vi "Unloading.vi"(8 "error In":errorcluster) -> (0 "error out":errorcluster)   [LabVIEW 2017]
uses:
  <vilib>/Utility/error.llb/DialogType.ctl
  Controls/Unloading_Cyc_Data.ctl
  Controls/QUEUE_STATES.ctl
  Controls/Unload_St.ctl
  <vilib>/Utility/file.llb/Read Delimited Spreadsheet (string).vi
  Global/PLC_to_Auto.vi
  <vilib>/Instr/_visa.llb/VISA Configure Serial Port (Instr).vi
panel:
  out "qr scanned":bool=TRUE
  out "SELECTED Chld Part":T1
  out "Expected Code:":string
  out "DOOR NO.":string
  out "output cluster":cluster{"Feeder Door Open":bool, "Address":u16}
  out "raw scan code":string
  in  "Boolean":bool
  in  "String":string
  out "Bins/Box":i32
  out "Scanner Comm":bool
  out "Stop scanner":bool
  out "CYCLE STATUS":string
  out "CURRENT PLAN":T2
  out "SCAN CODE:":string
  out "Selected Plan structure":string[][](table)
  out "Plan Selected:":string
  out "USER:-":string
  in  "Stop":bool
  out "DATE/TIME":string
  out "Screen Name":string
  # "DOOR NUMBER"
  # "BIN STATUS"
  # "DOOR NUMBER"
  # "BIN STATUS"
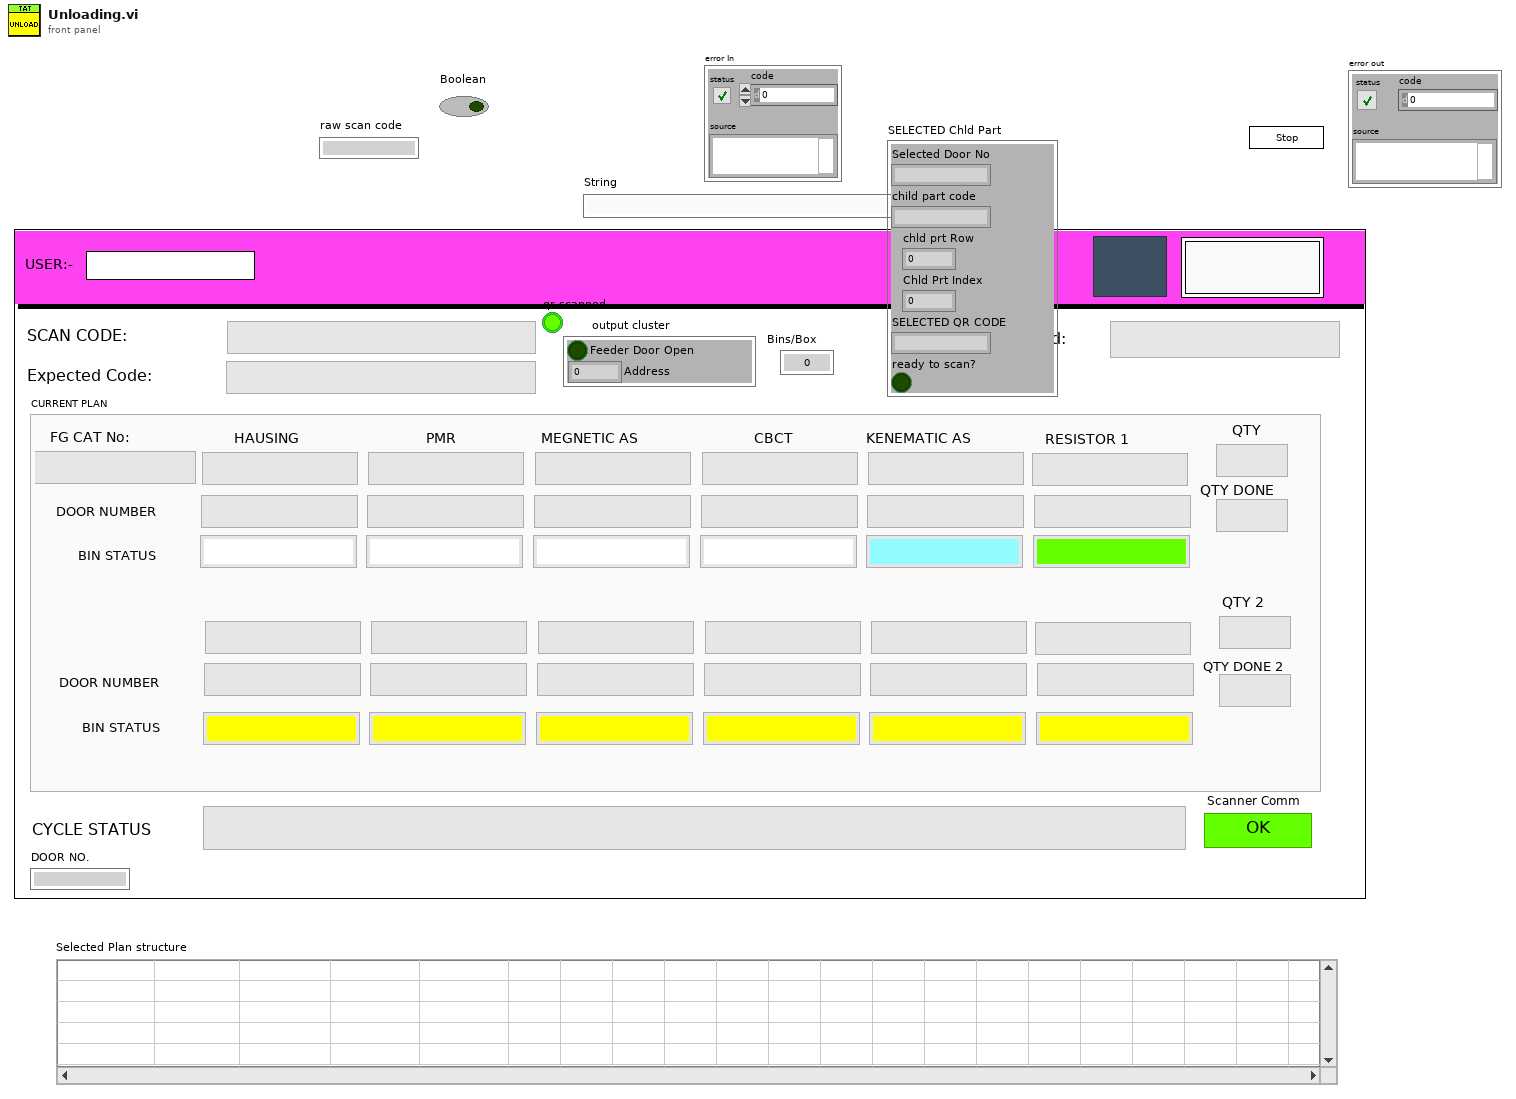
[diagram p1: front panel]
types:
  T1 = cluster{"Selected Door No":string, "child part code":string, "chld prt Row":i32, "Chld Prt Index":i32, "SELECTED QR CODE":string, "ready to scan?":bool}
  T2 = cluster{"FG CAT No:":string, "HAUSING":string, "PMR":string, "MEGNETIC AS":string, "CBCT":string, "KENEMATIC AS":string, "RESISTOR 1":string, "HAUSING DOOR":string, "PMR DOOR":string, "MAGNETIC AS DOOR":string, "CBCT DOOR":string, "KINEMATIC AS DOOR":string, "RESISTOR 1 DOOR":string, "HAUSING FEED STATUS":string, "PMR FEED STATUS":string, "MAGNETIC AS FEEED STATUS":string, "CBCT FEED STATUS":string, "KINEMATIC AS FEED STATUS":string, "RESISTOR 1 FEED STATUS":string, "QTY":string, "QTY DONE":string, "HAUSING 2":string, "PMR 2":string, "MEGNETIC AS 2":string, "CBCT 2":string, "KENEMATIC AS 2":string, "RESISTOR 2":string, "HAUSING DOOR 2":string, "PMR DOOR 2":string, "MAGNETIC AS DOOR 2":string, "CBCT DOOR 2":string, "KINEMATIC AS DOOR 2":string, "RESISTOR 1 DOOR 2":string, "HAUSING FEED STATUS 2":string, "PMR FEED STATUS 2":string, "MAGNETIC AS FEEED STATUS 2":string, "CBCT FEED STATUS 2":string, "KINEMATIC AS FEED STATUS 2":string, "RESISTOR 1 FEED STATUS 2":string, "QTY 2":string, "QTY DONE 2":string}
  T3 = typedef "Unloading_Cyc_Data.ctl" = cluster{"Cycle_Plan":path, "Plan_Data":string[][], "Scanned_Data":string[], "SELECTED Chld Part":cluster{"Selected Door No":string, "child part code":string, "chld prt Row":i32, "Chld Prt Index":i32, "EXPECTED QR CODE":string, "ready to scan?":bool}, "feed Status Indi":refnum<vi>[], "Recipe Selected":cluster{"Bin/Box Mode":i32, "Selected Section":i32}, "ALL CSV DATA":string[][]}
  T4 = typedef "DialogType.ctl" = u16
  T5 = enum32{"invalid app kind", "Development System", "Run Time System", "Student Edition", "Embedded LabVIEW", "Evaluation", "Custom"}
  T6 = typedef "QUEUE_STATES.ctl" = enum16{"CREATE Q", "EN Q", "DE Q", "CLOSE Q"}
  T7 = cluster{"Printer IP":string, "PLC IP Address":string, "Scanner Com":refnum<visa-resource-name>}
  T8 = typedef "Unload_St.ctl" = enum16{"Package_Qty_Count", "GENERATE_QR_PRNT", "Cluster_update", "Read_Plan", "QR_Scanned", "Int", "Chk_Previous_State", "Chk_Loaded_and_Open_Door", "Update_Plan_Cluster", "Error_Handler", "Wait", "Close_Door", "Stop"}
  T9 = cluster{"Selected Door No":string, "child part code":string, "chld prt Row":i32, "Chld Prt Index":i32, "EXPECTED QR CODE":string, "ready to scan?":bool}
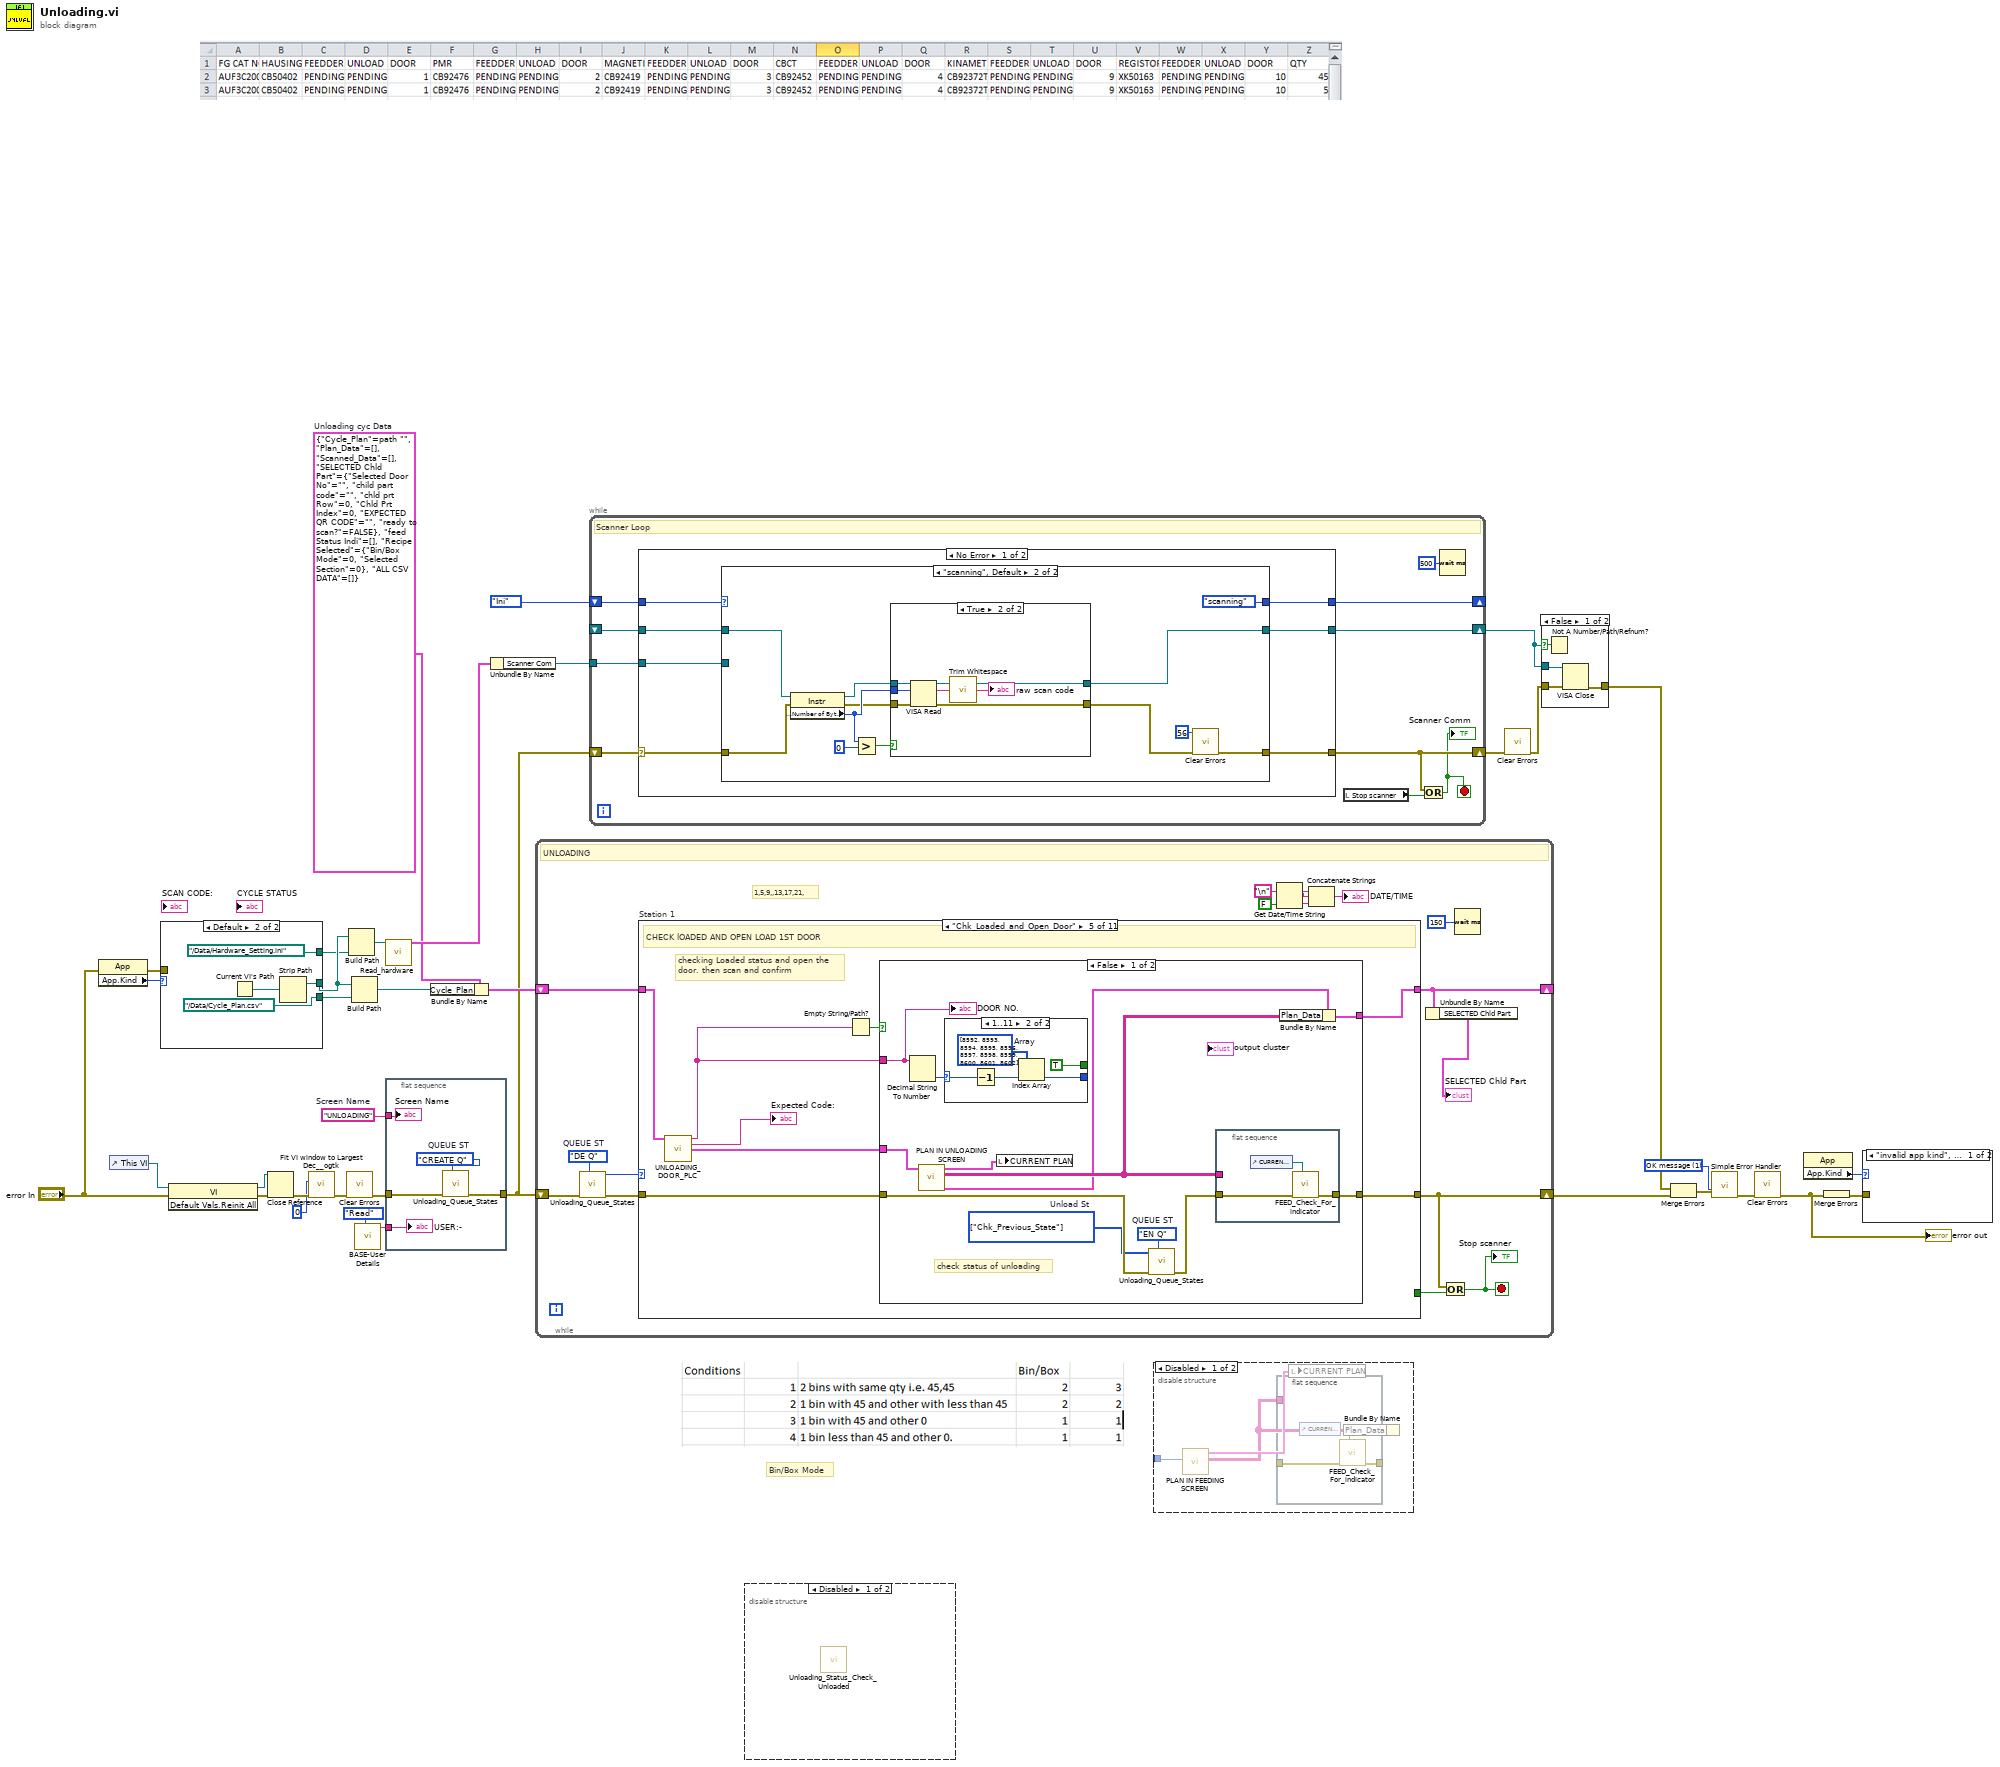
[diagram p0: block diagram]
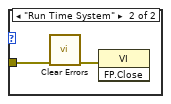
[diagram p3: hidden frame]
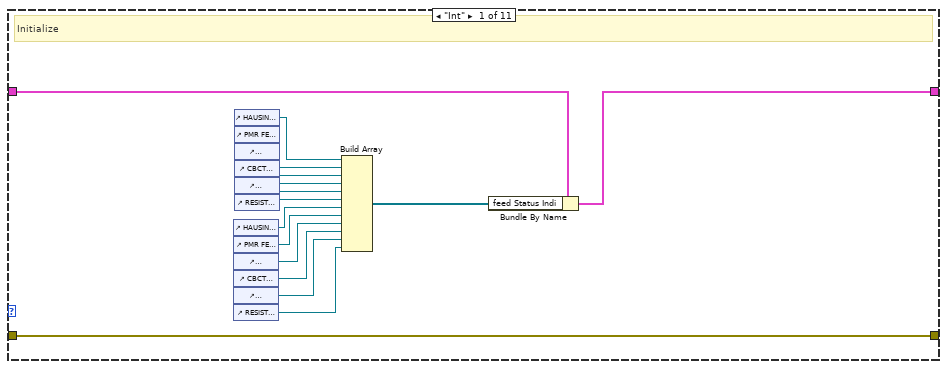
[diagram p4: hidden frame]
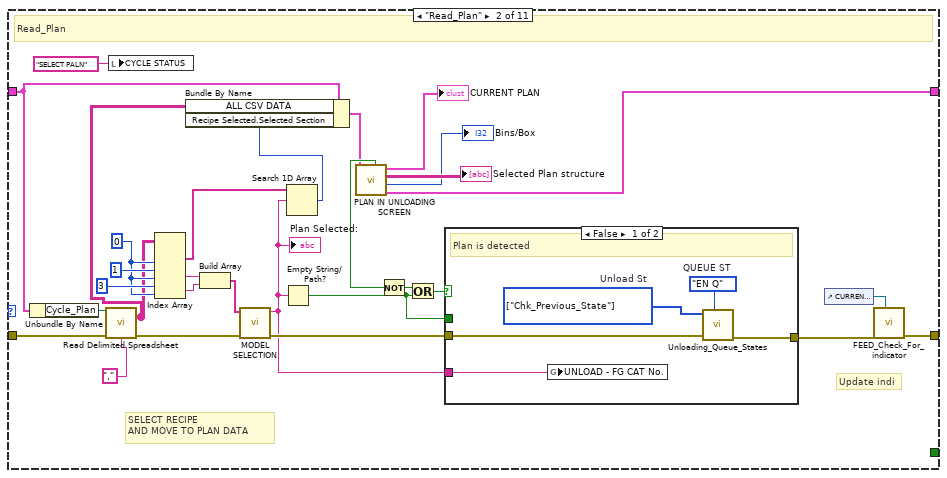
[diagram p5: hidden frame]
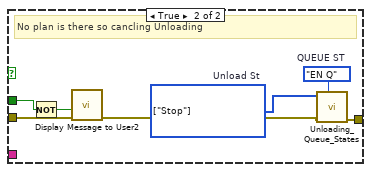
[diagram p6: hidden frame]
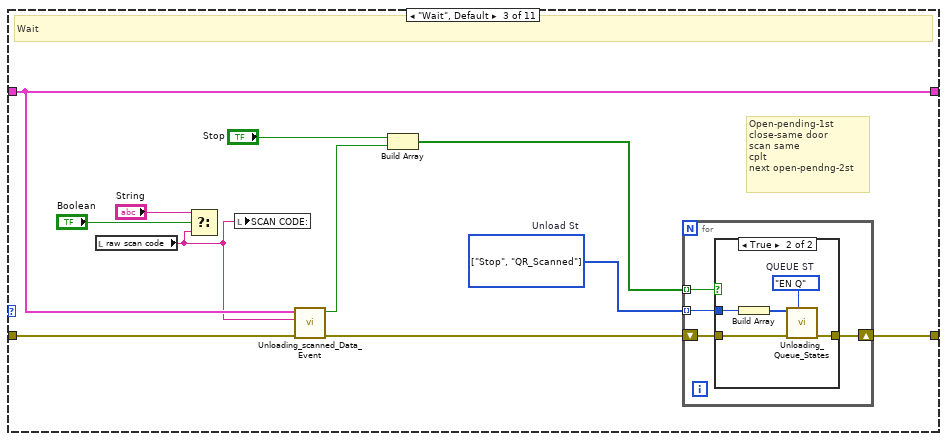
[diagram p7: hidden frame]
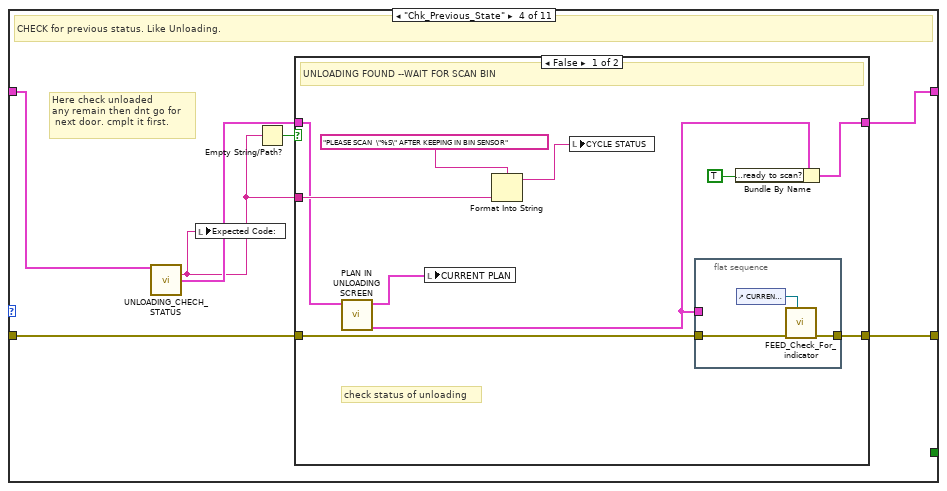
[diagram p9: hidden frame]
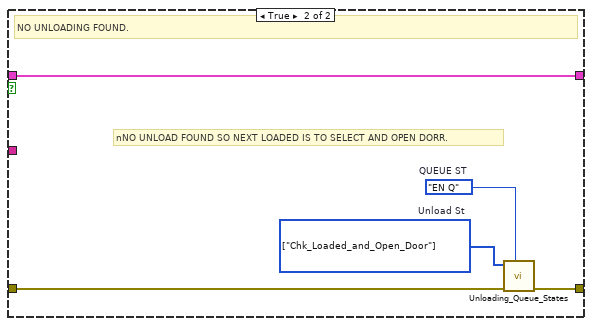
[diagram p10: hidden frame]
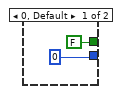
[diagram p11: hidden frame]
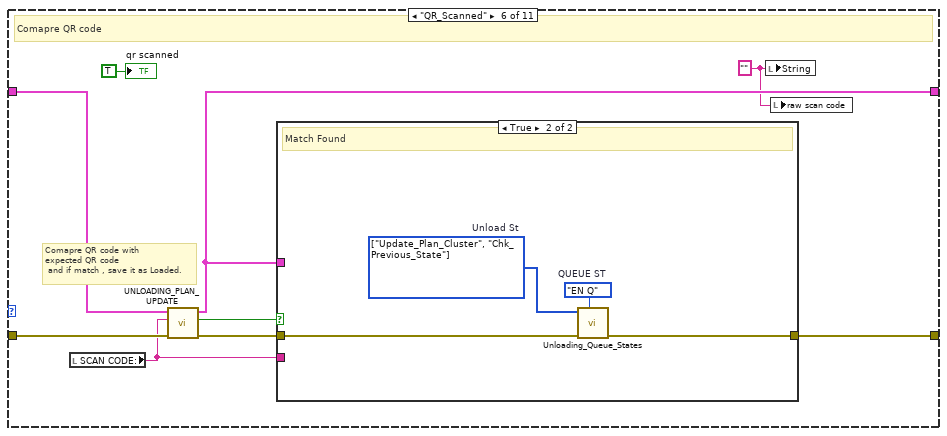
[diagram p13: hidden frame]
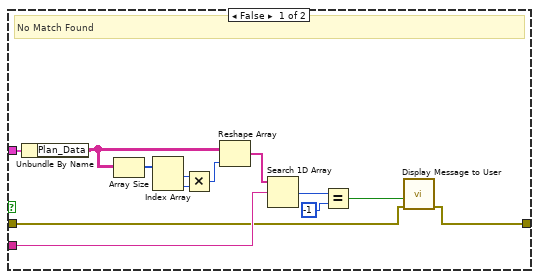
[diagram p14: hidden frame]
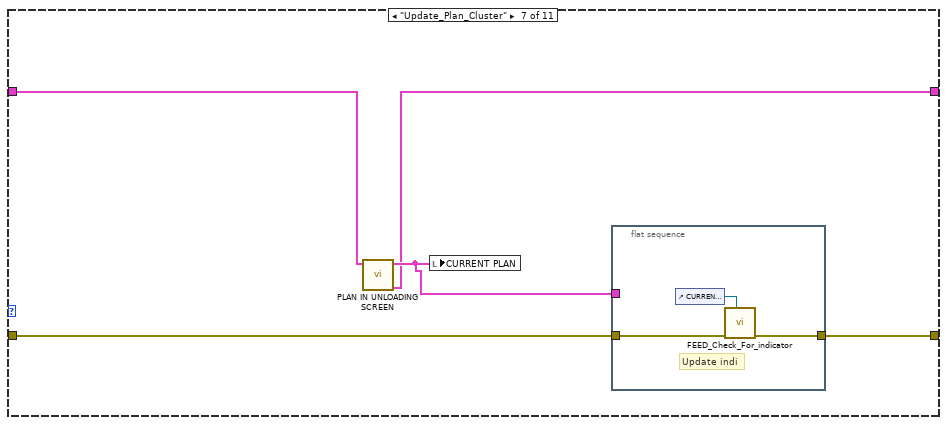
[diagram p15: hidden frame]
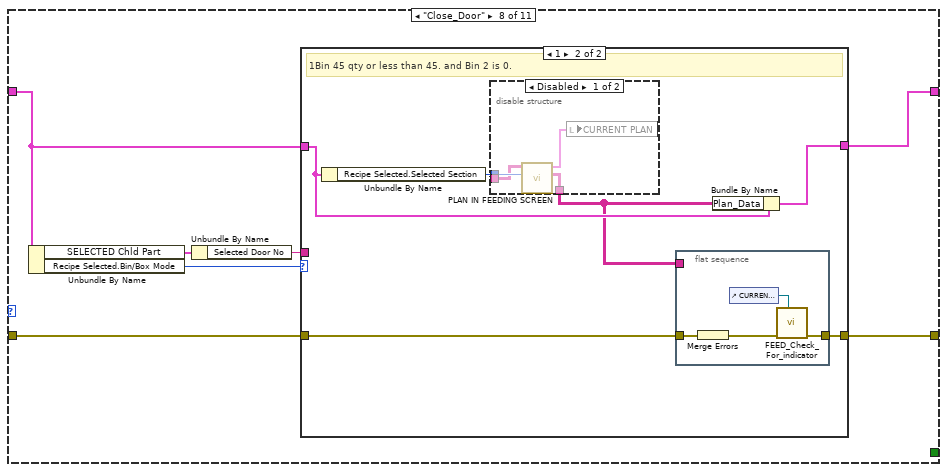
[diagram p16: hidden frame]
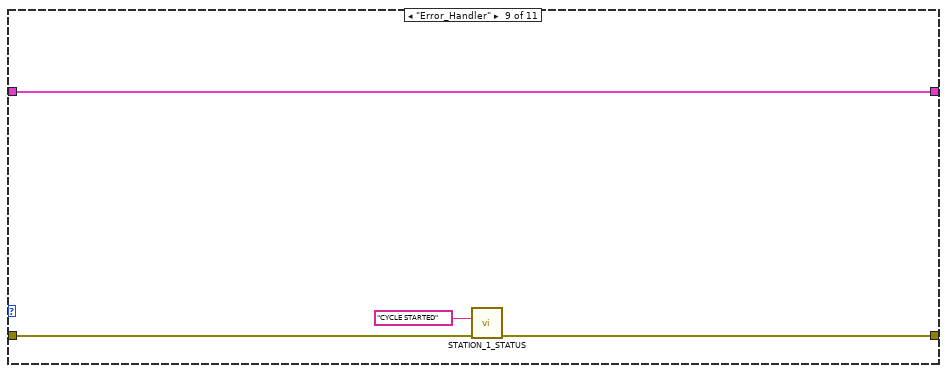
[diagram p19: hidden frame]
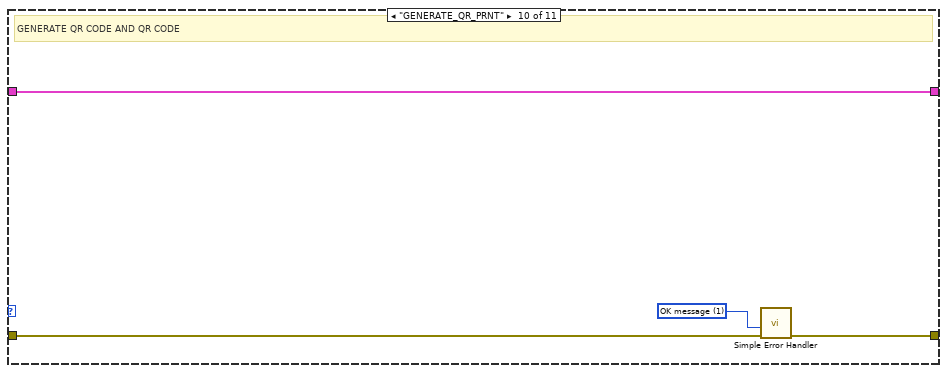
[diagram p20: hidden frame]
diagram:
  w1 = T3 {"Cycle_Plan"=path "", "Plan_Data"=[], "Scanned_Data"=[], "SELECTED Chld Part"={"Selected Door No"="", "child part code"="", "chld prt Row"=0, "Chld Prt Index"=0, "EXPECTED QR CODE"="", "ready to scan?"=FALSE}, "feed Status Indi"=[], "Recipe Selected"={"Bin/Box Mode"=0, "Selected Section"=0}, "ALL CSV DATA"=[]}  # Unloading cyc Data
  w18 = "UNLOADING"  # Screen Name
  w29 = T4 1 items=["no dialog", "OK message", "continue or stop message", "OK message + warnings", "continue/stop + warnings"] ("type of dialog (OK msg:1)")
  # "Bin/Box Mode"
  n1 = property class="App"(error in="error In") -> (error out=w25:errorcluster, "App.Kind"=w27:T5)  [unwired: 1 in, 1 out]
  n2 = control-ref of="This VI"() -> (w36:refnum<vi>)
  n3 = case shown="Default" w27 {
    tunnel: [path "Data/Cycle_Plan.csv" ("path") path "../Data/Cycle_Plan.csv" ("path")] -> w26
    tunnel: [w37 w41] -> w7
    tunnel: w25 -> [_ _]
    tunnel: [path "Data/Hardware_Setting.ini" ("path") path "../Data/Hardware_Setting.ini" ("path")] -> w6
    frame "Run Time System" {
      n4 = call <vilib>:"Application Directory.vi"() -> ("Application Directory"=w37:path)
    }
    frame Default {
      n5 = Current VI's Path() -> (path=w42:path)
      n6 = Strip Path(path=w42) -> (stripped path=w41:path)  [unwired: 1 out]
    }
  }
  n7 = invoke class="VI" method="Default Vals.Reinit All"(reference=w36, error in="error In") -> (reference out=w34:refnum<vi>, error out=w35:errorcluster)  [unwired: 1 in, 1 out]
  n8 = Close Reference(reference=w34, error in (no error)=w35) -> (error out=w33:errorcluster)
  n9 = call <userlib>:"Fit VI window to Largest Dec__ogtk.vi"("error in (no error)"=w33, "border spacing (2 px)"=0) -> ("error out"=w23:errorcluster)  [unwired: 4 in, 1 out]
  n10 = call <vilib>:"Clear Errors.vi"("error in (no error)"=w23) -> ("error out"=w11:errorcluster)  [unwired: 5 in, 1 out]
  n11 = Build Path(base path=w7, name or relative path=w6) -> (appended path=w5:path)
  n12 = Build Path(base path=w7, name or relative path=w26) -> (appended path=w20:path)
  n13 = call "BASE-User Details.vi"("Enum"=enum16{"Read", "Write"}."Read") -> ("User Name Out"=w30:string)  [unwired: 9 in, 1 out]
  n14 = flat-sequence {
    tunnel: [w45] -> w12
    tunnel: w11 -> [w46]
    tunnel: w30 -> [w48]
    tunnel: w18 -> [w47]
    frame #0 {
      w44 = QUEUE_STATES."CREATE Q"  # QUEUE ST
      n15 = call "Unloading_Queue_States.vi"("QUEUE ST"=w44, "error in"=w46) -> ("error OUT"=w45:errorcluster)  [unwired: 8 in, 1 out]
      "USER:-" <- w48
      "Screen Name" <- w47
    }
  }
  n16 = call "Read_hardware.vi"("configuration file path"=w5) -> ("data"=w9:T7)  [unwired: 10 in]
  n17 = Bundle By Name(cluster=w1, "Cycle_Plan"=w20) -> (w19:T3)
  n18 = Unbundle By Name(w9) -> ("Scanner Com"=w8:refnum<visa-resource-name>)
  n19 = while {
    shift-right: [w50] -> _
    shift-left: w19 -> [w57]
    shift-right: [w55] -> w10
    shift-left: w12 -> [w54]
    stop <- w56 stop-if-true
    w52 = QUEUE_STATES."DE Q"  # QUEUE ST
    # "1,5,9,,13,17,21,"
    # "UNLOADING"
    n20 = call "Unloading_Queue_States.vi"("QUEUE ST"=w52, "error in"=w54) -> ("error OUT"=w53:errorcluster, "Unload ST"=w51:T8)  [unwired: 8 in]
    n21 = case "Station 1" shown="\"Chk_Loaded_and_Open_Door\"" w51 {
      tunnel: [_ _ _ _ _ _ _ _ _ _ TRUE] -> w58
      tunnel: [w80 w97 w130 w148 w173 w205 w229 w239 w258 w263 w265] -> w55
      tunnel: w53 -> [w80 w108 w124 w147 w172 w208 w230 w240 w259 w262 w269]
      tunnel: w57 -> [w67 w82 w126 w143 w169 w207 w227 w236 w257 w261 w268]
      tunnel: [w66 w81 w126 w146 w170 w203 w226 w235 w257 w261 w268] -> w50
      frame "Int" {
        # "Initialize"
        n22 = control-ref of="HAUSING FEED STATUS 2"() -> (w74:refnum<vi>)
        n23 = control-ref of="PMR FEED STATUS 2"() -> (w75:refnum<vi>)
        n24 = control-ref of="MAGNETIC AS FEEED STATUS 2"() -> (w76:refnum<vi>)
        n25 = control-ref of="CBCT FEED STATUS 2"() -> (w77:refnum<vi>)
        n26 = control-ref of="KINEMATIC AS FEED STATUS 2"() -> (w78:refnum<vi>)
        n27 = control-ref of="RESISTOR 1 FEED STATUS 2"() -> (w79:refnum<vi>)
        n28 = control-ref of="HAUSING FEED STATUS"() -> (w68:refnum<vi>)
        n29 = control-ref of="PMR FEED STATUS"() -> (w69:refnum<vi>)
        n30 = control-ref of="MAGNETIC AS FEEED STATUS"() -> (w70:refnum<vi>)
        n31 = control-ref of="CBCT FEED STATUS"() -> (w71:refnum<vi>)
        n32 = control-ref of="KINEMATIC AS FEED STATUS"() -> (w72:refnum<vi>)
        n33 = control-ref of="RESISTOR 1 FEED STATUS"() -> (w73:refnum<vi>)
        n34 = Build Array(w68, w69, w70, w71, w72, w73, w74, w75, w76, w77, w78, w79) -> (w65:refnum<vi>[])
        n35 = Bundle By Name(cluster=w67, "feed Status Indi"=w65) -> (w66:T3)
      }
      frame "Read_Plan" {
        w100 = 0
        # "SELECT RECIPE\nAND MOVE TO PLAN DATA"
        # "Update indi"
        # "Read_Plan"
        n36 = Unbundle By Name(w82) -> ("Cycle_Plan"=w107:path)
        n37 = call-poly <vilib>:"Read Delimited Spreadsheet.vi"("file path (dialog if empty)"=w107, "error in (no error)"=w108, "delimiter (\\t)"=",") -> ("all rows"=w83:string[][], "error out"=w101:errorcluster)  [unwired: 7 in, 4 out]
        n38 = local write "CYCLE STATUS"("SELECT PALN") -> ()
        n39 = Index Array(array=w83, index (col) #1=w100, index (row) #2=1, index (col) #2=w100, index (row) #3=3, index (col) #3=w100) -> (element #1=w99:string[], element #2=w104:string, element #3=w103:string)  [unwired: 1 in]
        n40 = Build Array(w104, w103) -> (w102:string[])
        n41 = call "MODEL SELECTION.vi"("error in (no error)"=w101, "Plan List"=w102) -> ("error out 2"=w95:errorcluster, "Plan Selected"=w87:string)  [unwired: 7 in, 1 out]
        "Plan Selected:" <- w87
        n42 = Empty String/Path?(string/path=w87) -> (empty?=w91:bool)
        n43 = Search 1D Array(1D array=w99, element=w87) -> (index of element=w85:i32)  [unwired: 1 in]
        n44 = Bundle By Name(cluster=w82, "ALL CSV DATA"=w83, "Recipe Selected.Selected Section"=w85) -> (w84:T3)
        n45 = call "PLAN IN UNLOADING SCREEN.vi"("Unloading cyc Data"=w84) -> ("Unloading cyc Data 2"=w81:T3, "Bin/Box"=→"Bins/Box":i32, "PLAN DATA Out"=→"Selected Plan structure":string[][], "CURRENT PLAN"=→"CURRENT PLAN":T2, "FEED CMPLT?"=w93:bool)  [unwired: 6 in]
        n46 = Not(x=w93) -> (.not. x?=w92:bool)
        n47 = Or(x=w92, y=w91) -> (x .or. y?=w94:bool)
        n48 = case shown="False" w94 {
          tunnel: w95 -> [w114 w119]
          tunnel: [w113 w120] -> w98
          tunnel: w91 -> [_ w117]
          tunnel: w87 -> [w110 _]
          frame False {
            w111 = T8[] [enum."Chk_Previous_State"] items=["Package_Qty_Count", "GENERATE_QR_PRNT", "Cluster_update", "Read_Plan", "QR_Scanned", "Int", "Chk_Previous_State", "Chk_Loaded_and_Open_Door", "Update_Plan_Cluster", "Error_Handler", "Wait", "Close_Door", "Stop"]  # Unload St
            w112 = QUEUE_STATES."EN Q"  # QUEUE ST
            # "Plan is detected"
            n49 = global write "PLC_to_Auto.vi" "UNLOAD - FG CAT No."(w110) -> ()
            n50 = call "Unloading_Queue_States.vi"("QUEUE ST"=w112, "error in"=w114, "Unload St"=w111) -> ("error OUT"=w113:errorcluster)  [unwired: 7 in, 1 out]
          }
          frame True {
            w115 = T8[] [enum."Stop"] items=["Package_Qty_Count", "GENERATE_QR_PRNT", "Cluster_update", "Read_Plan", "QR_Scanned", "Int", "Chk_Previous_State", "Chk_Loaded_and_Open_Door", "Update_Plan_Cluster", "Error_Handler", "Wait", "Close_Door", "Stop"]  # Unload St
            w121 = QUEUE_STATES."EN Q"  # QUEUE ST
            # "No plan is there so cancling Unloading"
            n51 = Not(x=w117) -> (.not. x?=w116:bool)
            n52 = call "Display Message to User2"("error in (no error)"=w119, "Enable"=w116) -> ("error out"=w118:errorcluster)  [unwired: 8 in, 1 out]
            n53 = call "Unloading_Queue_States.vi"("QUEUE ST"=w121, "error in"=w118, "Unload St"=w115) -> ("error OUT"=w120:errorcluster)  [unwired: 7 in, 1 out]
          }
        }
        n54 = control-ref of="CURRENT PLAN"() -> (w96:refnum<vi>)
        n55 = call "FEED_Check_For_indicator.vi"("CURRENT PLAN"=w96, "error in (no error)"=w98) -> ("error out"=w97:errorcluster)  [unwired: 9 in]
      }
      frame "Wait", Default {
        w127 = T8[] [enum."Stop", enum."QR_Scanned"] items=["Package_Qty_Count", "GENERATE_QR_PRNT", "Cluster_update", "Read_Plan", "QR_Scanned", "Int", "Chk_Previous_State", "Chk_Loaded_and_Open_Door", "Update_Plan_Cluster", "Error_Handler", "Wait", "Close_Door", "Stop"]  # Unload St
        # "Open-pending-1st\nclose-same door\nscan same\ncplt\nnext open-pendng-2st"
        # "Wait"
        n56 = local read "raw scan code"() -> (w122:string)
        n57 = Select(t="String", s="Boolean", f=w122) -> ()  [unwired: 1 out]
        n58 = local write "SCAN CODE:"(w122) -> ()
        n59 = call "Unloading_scanned_Data_Event.vi"("Unloading cyc Data"=w126, "Scanned  Data"=w122, "error in"=w124) -> ("Scanned ?"=w125:bool, "error out"=w123:errorcluster)  [unwired: 6 in]
        n60 = Build Array("Stop", w125) -> (w128:bool[])
        n61 = for {
          shift-right: [w135] -> w130
          shift-left: w123 -> [w136]
          tunnel: w128 -> [w134] mode=indexing
          tunnel: w127 -> [w133] mode=indexing
          n62 = case shown="True" w134 {
            tunnel: w136 -> [w137 w141]
            tunnel: [w137 w140] -> w135
            tunnel: w133 -> [_ w139]
            frame False {
            }
            frame True {
              w142 = QUEUE_STATES."EN Q"  # QUEUE ST
              n63 = Build Array(w139) -> (w138:T8[])
              n64 = call "Unloading_Queue_States.vi"("QUEUE ST"=w142, "error in"=w141, "Unload St"=w138) -> ("error OUT"=w140:errorcluster)  [unwired: 7 in, 1 out]
            }
          }
        }
      }
      frame "Chk_Previous_State" {
        # "Here check unloaded\nany remain then dnt go for\n next door. cmplt it first."
        # "CHECK for previous status. Like Unloading."
        n65 = call "UNLOADING_CHECH_STATUS.vi"("Unloading cyc Data"=w143) -> ("QR Code"=w144:string, "Unloading cyc Data OUT"=w145:T3)  [unwired: 12 in, 1 out]
        n66 = local write "Expected Code:"(w144) -> ()
        n67 = Empty String/Path?(string/path=w144) -> (empty?=w149:bool)
        n68 = case shown="False" w149 {
          tunnel: [w158 w165] -> w148
          tunnel: w147 -> [w159 w166]
          tunnel: w145 -> [w150 w167]
          tunnel: [w156 w167] -> w146
          tunnel: w144 -> [w154 _]
          frame False {
            # "check status of unloading"
            # "UNLOADING FOUND --WAIT FOR SCAN BIN"
            n69 = call "PLAN IN UNLOADING SCREEN.vi"("Unloading cyc Data"=w150) -> ("Unloading cyc Data 2"=w151:T3, "CURRENT PLAN"=w157:T2)  [unwired: 6 in, 3 out]
            n70 = local write "CURRENT PLAN"(w157) -> ()
            n71 = Format Into String(format string="PLEASE SCAN  \"%S\" AFTER KEEPING IN BIN SENSOR", w154) -> (resulting string=w153:string)  [unwired: 2 in, 1 out]
            n72 = local write "CYCLE STATUS"(w153) -> ()
            n73 = flat-sequence {
              tunnel: w159 -> [w161]
              tunnel: [w160] -> w158
              tunnel: w151 -> [_]
              frame #0 {
                n74 = control-ref of="CURRENT PLAN"() -> (w162:refnum<vi>)
                n75 = call "FEED_Check_For_indicator.vi"("CURRENT PLAN"=w162, "error in (no error)"=w161) -> ("error out"=w160:errorcluster)  [unwired: 9 in]
              }
            }
            n76 = Bundle By Name(cluster=w151, "SELECTED Chld Part.ready to scan?"=TRUE) -> (w156:T3)
          }
          frame True {
            w163 = T8[] [enum."Chk_Loaded_and_Open_Door"] items=["Package_Qty_Count", "GENERATE_QR_PRNT", "Cluster_update", "Read_Plan", "QR_Scanned", "Int", "Chk_Previous_State", "Chk_Loaded_and_Open_Door", "Update_Plan_Cluster", "Error_Handler", "Wait", "Close_Door", "Stop"]  # Unload St
            w164 = QUEUE_STATES."EN Q"  # QUEUE ST
            # "nNO UNLOAD FOUND SO NEXT LOADED IS TO SELECT AND OPEN DORR."
            # "NO UNLOADING FOUND."
            n77 = call "Unloading_Queue_States.vi"("QUEUE ST"=w164, "error in"=w166, "Unload St"=w163) -> ("error OUT"=w165:errorcluster)  [unwired: 7 in, 1 out]
          }
        }
      }
      frame "Chk_Loaded_and_Open_Door" {
        # "checking Loaded status and open the\ndoor. then scan and confirm"
        # "CHECK lOADED AND OPEN LOAD 1ST DOOR"
        n78 = call "UNLOADING_DOOR_PLC.vi"("Unloading cyc Data"=w169) -> ("DOOR NO."=w175:string, "QR Code"=→"Expected Code:":string, "Unloading cyc Data 2"=w168:T3)  [unwired: 11 in, 1 out]
        n79 = Empty String/Path?(string/path=w175) -> (empty?=w174:bool)
        n80 = case shown="False" w174 {
          tunnel: w175 -> [w186 _]
          tunnel: [w185 w199] -> w173
          tunnel: w172 -> [w179 w199]
          tunnel: [w182 w198] -> w170
          tunnel: w168 -> [w181 w198]
          frame False {
            w177 = T8[] [enum."Chk_Previous_State"] items=["Package_Qty_Count", "GENERATE_QR_PRNT", "Cluster_update", "Read_Plan", "QR_Scanned", "Int", "Chk_Previous_State", "Chk_Loaded_and_Open_Door", "Update_Plan_Cluster", "Error_Handler", "Wait", "Close_Door", "Stop"]  # Unload St
            w180 = QUEUE_STATES."EN Q"  # QUEUE ST
            # "check status of unloading"
            n81 = Decimal String To Number(string=w186) -> (number=w187:i32)  [unwired: 2 in, 1 out]
            n82 = call "PLAN IN UNLOADING SCREEN.vi"("Unloading cyc Data"=w181) -> ("Unloading cyc Data 2"=w176:T3, "PLAN DATA Out"=w183:string[][], "CURRENT PLAN"=w184:T2)  [unwired: 6 in, 2 out]
            n83 = case shown="1..11" w187 {
              selector: w187 -> [_ w197]
              tunnel: [u16 0 w196] -> _
              tunnel: [FALSE TRUE] -> _
              frame 0, Default {
              }
              frame 1..11 {
                w194 = i32[] [8592, 8593, 8594, 8595, 8596, 8597, 8598, 8599, 8600, 8601, 8602]  # Array
                n84 = Decrement(x=w197) -> (x-1=w193:i32)
                n85 = Index Array(array=w194, index=w193) -> (element=w196:i32)
              }
            }
            n86 = local write "CURRENT PLAN"(w184) -> ()
            n87 = call "Unloading_Queue_States.vi"("QUEUE ST"=w180, "error in"=w179, "Unload St"=w177) -> ("error OUT"=w178:errorcluster)  [unwired: 7 in, 1 out]
            n88 = flat-sequence {
              tunnel: w178 -> [w189]
              tunnel: [w188] -> w185
              tunnel: w183 -> [_]
              frame #0 {
                n89 = control-ref of="CURRENT PLAN"() -> (w190:refnum<vi>)
                n90 = call "FEED_Check_For_indicator.vi"("CURRENT PLAN"=w190, "error in (no error)"=w189) -> ("error out"=w188:errorcluster)  [unwired: 9 in]
              }
            }
            n91 = Bundle By Name(cluster=w176, "Plan_Data"=w183) -> (w182:T3)
            "DOOR NO." <- w186
          }
          frame True {
          }
        }
      }
      frame "QR_Scanned" {
        w200 = ""
        # "Comapre QR code with \nexpected QR code\n and if match , save it as Loaded."
        # "Comapre QR code"
        n92 = local read "SCAN CODE:"() -> (w202:string)
        n93 = call "UNLOADING_PLAN_UPDATE.vi"("error in (no error)"=w208, "SCAN CODE:"=w202, "Unloading cyc Data in"=w207) -> ("error out"=w206:errorcluster, "QR Match ?"=w204:bool, "Unloading cyc Data out"=w203:T3)  [unwired: 6 in]
        n94 = case shown="True" w204 {
          tunnel: w206 -> [w210 w224]
          tunnel: [w209 w223] -> w205
          tunnel: w203 -> [w221 _]
          tunnel: w202 -> [w214 _]
          frame False {
            # "No Match Found"
            n95 = Unbundle By Name(w221) -> ("Plan_Data"=w216:string[][])
            n96 = Array Size(array=w216) -> (size(s)=w220:i32[])
            n97 = Index Array(array=w220) -> (element #1=w218:i32, element #2=w219:i32)  [unwired: 2 in]
            n98 = Multiply(x=w218, y=w219) -> (x*y=w217:i32)
            n99 = Reshape Array(w216, w217) -> (w215:string[])
            n100 = Search 1D Array(1D array=w215, element=w214) -> (index of element=w213:i32)  [unwired: 1 in]
            n101 = Equal?(x=w213, y=-1) -> (x = y?=w211:bool)
            n102 = call "Display Message to User"("error in (no error)"=w210, "Enable"=w211) -> ("error out"=w209:errorcluster)  [unwired: 8 in, 1 out]
          }
          frame True {
            w222 = T8[] [enum."Update_Plan_Cluster", enum."Chk_Previous_State"] items=["Package_Qty_Count", "GENERATE_QR_PRNT", "Cluster_update", "Read_Plan", "QR_Scanned", "Int", "Chk_Previous_State", "Chk_Loaded_and_Open_Door", "Update_Plan_Cluster", "Error_Handler", "Wait", "Close_Door", "Stop"]  # Unload St
            w225 = QUEUE_STATES."EN Q"  # QUEUE ST
            # "Match Found"
            n103 = call "Unloading_Queue_States.vi"("QUEUE ST"=w225, "error in"=w224, "Unload St"=w222) -> ("error OUT"=w223:errorcluster)  [unwired: 7 in, 1 out]
          }
        }
        n104 = local write "String"(w200) -> ()
        n105 = local write "raw scan code"(w200) -> ()
        "qr scanned" <- TRUE
      }
      frame "Update_Plan_Cluster" {
        n106 = call "PLAN IN UNLOADING SCREEN.vi"("Unloading cyc Data"=w227) -> ("Unloading cyc Data 2"=w226:T3, "CURRENT PLAN"=w228:T2)  [unwired: 6 in, 3 out]
        n107 = local write "CURRENT PLAN"(w228) -> ()
        n108 = flat-sequence {
          tunnel: w230 -> [w232]
          tunnel: [w231] -> w229
          tunnel: w228 -> [_]
          frame #0 {
            # "Update indi"
            n109 = control-ref of="CURRENT PLAN"() -> (w233:refnum<vi>)
            n110 = call "FEED_Check_For_indicator.vi"("CURRENT PLAN"=w233, "error in (no error)"=w232) -> ("error out"=w231:errorcluster)  [unwired: 9 in]
          }
        }
      }
      frame "Close_Door" {
        n111 = Unbundle By Name(w236) -> ("SELECTED Chld Part"=w237:T9, "Recipe Selected.Bin/Box Mode"=w234:i32)
        n112 = Unbundle By Name(w237) -> ("Selected Door No"=w238:string)
        n113 = case shown="1" w234 {
          tunnel: w240 -> [w241 w248]
          tunnel: [w241 w245] -> w239
          tunnel: w238 -> [_ _]
          tunnel: w236 -> [w242 w246]
          tunnel: [w242 w243] -> w235
          frame 0, Default {
          }
          frame 1 {
            # "1Bin 45 qty or less than 45. and Bin 2 is 0."
            n114 = Unbundle By Name(w246) -> ("Recipe Selected.Selected Section"=w247:i32)
            n115 = disable-structure shown="Disabled" {
              disable-tunnel: w247 -> [w252 _]
              disable-tunnel: _ -> [w250 _]
              disable-tunnel: [w249 _] -> w244
              frame Disabled {
                n116 = call "PLAN IN FEEDING SCREEN.vi"("Section selected"=w252, "PLAN In"=w250) -> ("PLAN Out"=w249:string[][], "CURRENT PLAN"=w251:T2)  [unwired: 6 in, 2 out]
                n117 = local write "CURRENT PLAN"(w251) -> ()
              }
              frame Enabled {
              }
            }
            n118 = flat-sequence {
              tunnel: w248 -> [w256]
              tunnel: [w253] -> w245
              tunnel: w244 -> [_]
              frame #0 {
                n119 = Merge Errors(w256) -> (w254:errorcluster)
                n120 = control-ref of="CURRENT PLAN"() -> (w255:refnum<vi>)
                n121 = call "FEED_Check_For_indicator.vi"("CURRENT PLAN"=w255, "error in (no error)"=w254) -> ("error out"=w253:errorcluster)  [unwired: 9 in]
              }
            }
            n122 = Bundle By Name(cluster=w246, "Plan_Data"=w244) -> (w243:T3)
          }
        }
      }
      frame "Error_Handler" {
        n123 = call "STATION_1_STATUS.vi"("error in (no error)"=w259, "STATUS"="CYCLE STARTED" ("Cycle Status")) -> ("error out"=w258:errorcluster)  [unwired: 9 in]
      }
      frame "GENERATE_QR_PRNT" {
        w264 = T4 1 items=["no dialog", "OK message", "continue or stop message", "OK message + warnings", "continue/stop + warnings"] ("type of dialog (OK msg:1)")
        # "GENERATE QR CODE AND QR CODE"
        n124 = call <vilib>:"Simple Error Handler.vi"("type of dialog (OK msg:1)"=w264, "error in (no error)"=w262) -> ("error out"=w263:errorcluster)  [unwired: 3 in, 4 out]
      }
      frame "Stop" {
        w267 = QUEUE_STATES."CLOSE Q"  # QUEUE ST
        n125 = disable-structure shown="Disabled" {
          disable-tunnel: w269 -> [w272 _]
          disable-tunnel: [w271 _] -> w266
          frame Disabled {
            n126 = call "STATION_1_STATUS.vi"("error in (no error)"=w272, "STATUS"="STOP" ("Cycle Status")) -> ("error out"=w271:errorcluster)  [unwired: 9 in]
          }
          frame Enabled {
          }
        }
        n127 = call "Unloading_Queue_States.vi"("QUEUE ST"=w267, "error in"=w266) -> ("error OUT"=w265:errorcluster)  [unwired: 8 in, 1 out]
      }
    }
    n128 = Get Date/Time String(want seconds? (F)=FALSE) -> (date string=w62:string, time string=w61:string)  [unwired: 2 in]
    n129 = Concatenate Strings(w62, "\n", w61) -> (→"DATE/TIME":string)
    n130 = Unbundle By Name(w50) -> ("SELECTED Chld Part"=→"SELECTED Chld Part":T9)
    n131 = Or(x=w55, y=w58) -> (x .or. y?=w56:bool)
    "Stop scanner" <- w56
    n132 = Wait (ms)(milliseconds to wait=u32 150) -> ()  [unwired: 1 out]
  }
  n133 = while {
    shift-right: [w282] -> w16
    shift-left: w12 -> [w283]
    shift-right: [w280] -> _
    shift-left: enum16{"Ini", "scanning", "Close"}."Ini" -> [w281]
    tunnel: w8 -> [w279]
    shift-right: [w278] -> w13
    shift-left: _ -> [w277]
    stop <- w276 stop-if-true
    # "Scanner Loop"
    n134 = case shown="No Error" w283 {
      selector: w283 -> [w290 w320]
      tunnel: [w289 w319] -> w282
      tunnel: w281 -> [w288 _]
      tunnel: [w287 enum16{"Ini", "scanning", "Close"}."scanning"] -> w280
      tunnel: w279 -> [w286 _]
      tunnel: [w285 w317] -> w278
      tunnel: w277 -> [w284 w317]
      frame No Error {
        n135 = case shown="\"scanning\", Default" w288 {
          tunnel: w290 -> [w294 w298]
          tunnel: [w293 w306] -> w289
          tunnel: [enum16{"Ini", "scanning", "Close"}."scanning" enum16{"Ini", "scanning", "Close"}."scanning"] -> w287
          tunnel: w286 -> [w292 _]
          tunnel: [w291 w296] -> w285
          tunnel: w284 -> [_ w299]
          frame "Ini" {
            n136 = call-poly "VISA Configure Serial Port"("VISA resource name"=w292, "error in (no error)"=w294) -> ("VISA resource name out"=w291:refnum<visa-resource-name>, "error out"=w293:errorcluster)  [unwired: 12 in]
          }
          frame "scanning", Default {
            n137 = property class="Instr"(reference=w299, error in=w298) -> (reference out=w301:refnum<visa-resource-name>, error out=w302:errorcluster, "Serial Settings:Number of Bytes at Serial Port"=w303:u32)
            n138 = Greater?(x=w303, y=u32 0) -> (0:w304:bool)
            n139 = case shown="True" w304 {
              tunnel: w301 -> [w309 w316]
              tunnel: w302 -> [w308 w315]
              tunnel: w303 -> [_ w314]
              tunnel: [w309 w313] -> w296
              tunnel: [w308 w311] -> w297
              frame False {
              }
              frame True {
                n140 = VISA Read(VISA resource name=w316, byte count=w314, error in (no error)=w315) -> (VISA resource name out=w313:refnum<visa-resource-name>, read buffer=w312:string, error out=w311:errorcluster)  [unwired: 1 out]
                n141 = call <vilib>:"Trim Whitespace.vi"("string"=w312) -> ("trimmed string"=→"raw scan code":string)  [unwired: 1 in]
              }
            }
            n142 = call <vilib>:"Clear Errors.vi"("error in (no error)"=w297, "specific error code to clear (0: all)"=56) -> ("error out"=w306:errorcluster)  [unwired: 4 in, 1 out]
          }
        }
      }
      frame Error {
        n143 = Unbundle By Name(w320) -> ("code"=w321:i32)
        n144 = case shown="1" w321 {
          tunnel: w320 -> [w325 w327]
          tunnel: [w323 w326] -> w319
          frame 0, Default {
            w322 = T4 2 items=["no dialog", "OK message", "continue or stop message", "OK message + warnings", "continue/stop + warnings"] ("type of dialog (OK msg:1)")
            n145 = call <vilib>:"Simple Error Handler.vi"("type of dialog (OK msg:1)"=w322, "error in (no error)"=w325) -> ("error out"=w324:errorcluster)  [unwired: 3 in, 4 out]
            n146 = call <vilib>:"Clear Errors.vi"("error in (no error)"=w324) -> ("error out"=w323:errorcluster)  [unwired: 5 in, 1 out]
          }
          frame 1 {
            w328 = "THIS ERROR OCCURED AS SCREEN 1 IS NOT CONNECTED OR OFF"  # source
            # "Monitor not present/Off/disconnected"
            n147 = Bundle By Name(cluster=w327, "source"=w328) -> (w326:errorcluster)
          }
        }
      }
    }
    n148 = local read "Stop scanner"() -> (w274:bool)
    n149 = Or(x=w282, y=w274) -> (x .or. y?=w276:bool)
    "Scanner Comm" <- w276
    n150 = Wait (ms)(milliseconds to wait=u32 500) -> ()  [unwired: 1 out]
  }
  n151 = disable-structure shown="Disabled" {
    frame Disabled {
      n152 = call "Unloading_Status_Check_Unloaded.vi"() -> ()  [unwired: 11 in, 1 out]
    }
    frame Enabled {
    }
  }
  n153 = disable-structure shown="Disabled" {
    disable-tunnel: _ -> [w329 _]
    frame Disabled {
      n154 = call "PLAN IN FEEDING SCREEN.vi"("Section selected"=w329) -> ("PLAN Out"=w330:string[][], "CURRENT PLAN"=w331:T2)  [unwired: 7 in, 2 out]
      n155 = flat-sequence {
        tunnel: _ -> [w334]
        tunnel: [w333] -> _
        tunnel: w330 -> [_]
        frame #0 {
          n156 = control-ref of="CURRENT PLAN"() -> (w332:refnum<vi>)
          n157 = call "FEED_Check_For_indicator.vi"("CURRENT PLAN"=w332, "error in (no error)"=w334) -> ("error out"=w333:errorcluster)  [unwired: 9 in]
        }
      }
      n158 = local write "CURRENT PLAN"(w331) -> ()
      n159 = Bundle By Name("Plan_Data"=w330) -> ()  [unwired: 1 in, 1 out]
    }
    frame Enabled {
    }
  }
  n160 = call <vilib>:"Clear Errors.vi"("error in (no error)"=w16) -> ("error out"=w14:errorcluster)  [unwired: 5 in, 1 out]
  n161 = Not A Number/Path/Refnum?(number/path/refnum=w13) -> (NaN/Path/Refnum?=w15:bool)
  n162 = case shown="False" w15 {
    tunnel: w14 -> [w337 w338]
    tunnel: w13 -> [w335 _]
    tunnel: [w336 w338] -> w4
    frame False {
      n163 = VISA Close(VISA resource name=w335, error in (no error)=w337) -> (error out=w336:errorcluster)
    }
    frame True {
    }
  }
  n164 = Merge Errors(w4, w10) -> (w32:errorcluster)
  n165 = call <vilib>:"Simple Error Handler.vi"("type of dialog (OK msg:1)"=w29, "error in (no error)"=w32) -> ("error out"=w3:errorcluster)  [unwired: 3 in, 4 out]
  n166 = call <vilib>:"Clear Errors.vi"("error in (no error)"=w3) -> ("error out"=w2:errorcluster)  [unwired: 5 in, 1 out]
  "error out" <- w2
  n167 = property class="App"() -> ("App.Kind"=w28:T5)  [unwired: 2 in, 2 out]
  n168 = Merge Errors(w2) -> (w21:errorcluster)
  n169 = case shown="\"invalid app kind\", Default" w28 {
    tunnel: w21 -> [_ w340]
    frame "invalid app kind", Default {
    }
    frame "Run Time System" {
      n170 = call <vilib>:"Clear Errors.vi"("error in (no error)"=w340) -> ("error out"=w339:errorcluster)  [unwired: 5 in, 1 out]
      n171 = invoke class="VI" method="FP.Close"(error in=w339) -> ()  [unwired: 2 in, 3 out]
    }
  }
